vi "DAQ_Configure_it_live.vi"(0 "Pixel_clock_Hz":dbl, 1 "i(t)_block_size":i32, 2 "Position_X (µm)":dbl, 3 "Position_Y (µm)":dbl, 4 "Calib_X":dbl, 5 "Calib_Y":dbl, 7 "error in":errorcluster caption="entrée d'erreur", 8 "Device name":string) -> (22 "AO task":refnum<k21>, 24 "AI task":refnum<k21> caption="Ai task", 27 "error out":errorcluster caption="sortie d'erreur")   [LabVIEW 2026]
uses:
  <vilib>/DAQmx/write.llb/DAQmx Write (Analog 1D DBL NChan 1Samp).vi
  <vilib>/DAQmx/create/channels.llb/DAQmx Create Channel (AO-Voltage-Basic).vi
  <vilib>/DAQmx/miscellaneous.llb/DAQmx Fill In Error Info.vi
  <vilib>/DAQmx/create/channels.llb/DAQmx Create Channel (AI-Voltage-Basic).vi
  <vilib>/DAQmx/configure/timing.llb/DAQmx Timing (Sample Clock).vi
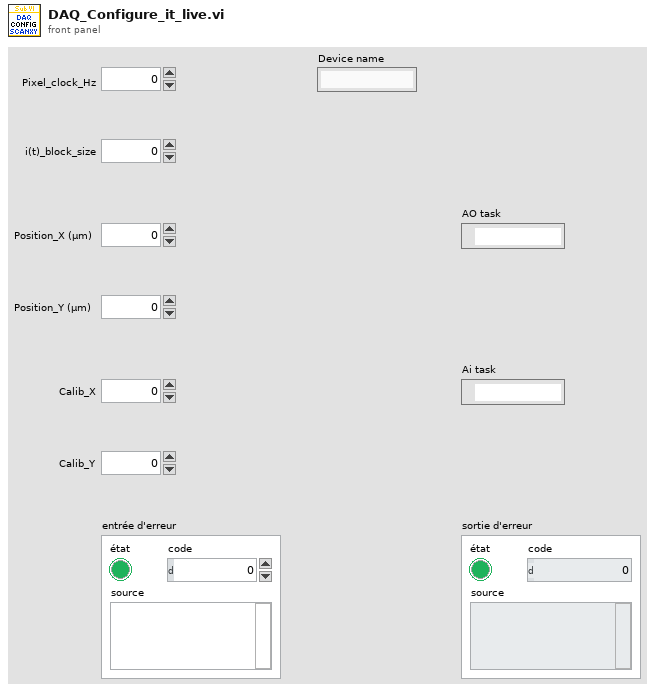
[diagram p1: front panel]
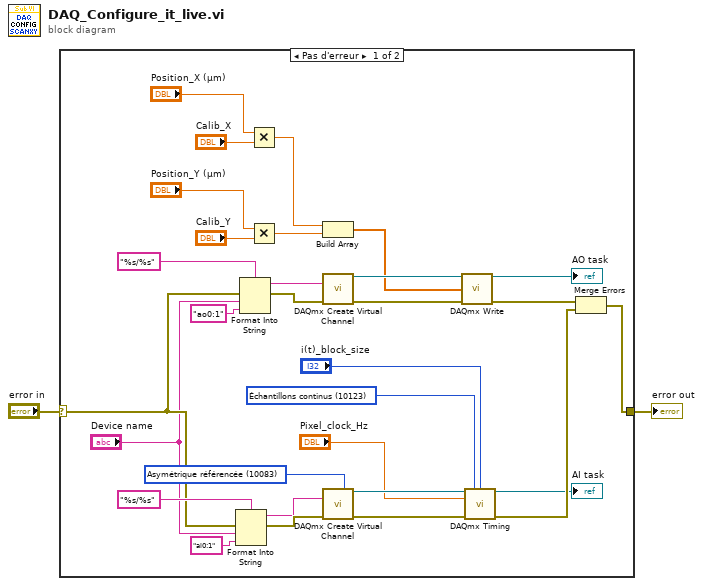
[diagram p0: block diagram]
diagram:
  n1 = case shown="Pas d'erreur" "error in" {
    selector: "error in" -> [w27 w33]
    tunnel: [w30 w33] -> w1
    frame No Error {
      w8 = 10123 items=["Échantillons finis"=10178, "Échantillons continus"=10123, "Point par point avec cadencement matériel"=12522] ("sample mode")
      w12 = 10083 items=["Par défaut"=-1, "Asymétrique référencée"=10083, "Asymétrique non référencée"=10078, "Différentielle"=10106, "Pseudodifférentielle"=12529] ("input terminal configuration")
      n2 = Format Into String(format string="%s/%s" ("chaîne de format"), error in=w27, "Device name", "ai0:1" ("entrée 2")) -> (resulting string=w13:string, error out=w14:errorcluster)  [unwired: 1 in]
      n3 = Format Into String(format string="%s/%s" ("chaîne de format"), error in=w27, "Device name", "ao0:1" ("entrée 2")) -> (resulting string=w25:string, error out=w24:errorcluster)  [unwired: 1 in]
      n4 = Multiply(x="Position_X (µm)", y="Calib_X") -> (x*y=w19:dbl)
      n5 = Multiply(x="Position_Y (µm)", y="Calib_Y") -> (x*y=w18:dbl)
      n6 = Build Array(w19, w18) -> (w17:dbl[])
      n7 = call-poly <vilib>:"DAQmx Create Virtual Channel.vi"("physical channels"=w25, "error in"=w24) -> ("task out"=w22:refnum<k21>, "error out"=w23:errorcluster)  [unwired: 12 in]
      n8 = call-poly <vilib>:"DAQmx Create Virtual Channel.vi"("input terminal configuration"=w12, "physical channels"=w13, "error in"=w14) -> ("task out"=w11:refnum<k21>, "error out"=w10:errorcluster)  [unwired: 11 in]
      n9 = call-poly <vilib>:"DAQmx Write.vi"("task/channels in"=w22, "data"=w17, "error in"=w23) -> ("task out"=→"AO task":refnum<k21>, "error out"=w5:errorcluster)  [unwired: 10 in, 1 out]
      n10 = call-poly <vilib>:"DAQmx Timing.vi"("task/channels in"=w11, "sample mode"=w8, "samples per channel"="i(t)_block_size", "rate"="Pixel_clock_Hz", "error in"=w10) -> ("task out"=→"AI task":refnum<k21>, "error out"=w6:errorcluster)  [unwired: 9 in]
      n11 = Merge Errors(w5, w6) -> (w30:errorcluster)
    }
    frame Error {
    }
  }
  "error out" <- w1
